vi "FGV_OBJ_error_buffer.vi"(4 "main_tab":refnum<vi>, 6 "thread":T1, 7 "option":T2=enum."display", 8 "error_in":errorcluster, 9 "error_indicator_global":refnum<vi>, 10 "error_indicator_tab":refnum<vi>, 11 "error_display_ref":refnum<vi>) -> (0 "error_out":errorcluster, 3 "error?":bool)   [LabVIEW 2020]
doc: "This VI check if error on error_in input is already in the buffer, and if not adds it to buffer and sends error event to event structure. VI also clears errors."
uses:
  FGV_OBJ_error_buffer.ctl
  MAIN/OBJ_thread.ctl
  <vilib>/Utility/miscctls.llb/LVRowAndColumnTypeDef.ctl
  <vilib>/Utility/miscctls.llb/LVRowAndColumnUnsignedTypeDef.ctl
  tristate_indicator_OBJ_test/FGV_tristate_indicator_OBJ_test.ctl
  _misc/AULocalize/SubVIs/Get Localized Phrase Compact Interface 1D.vi
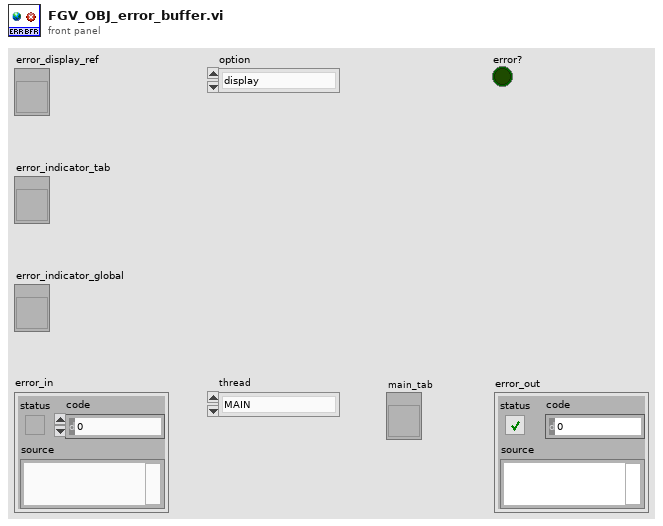
[diagram p1: front panel]
types:
  T1 = typedef "OBJ_thread.ctl" = enum16{"MAIN", "SCANNER", "MD - LEFT", "MD - RIGHT", "GUI TIMER"}
  T2 = typedef "FGV_OBJ_error_buffer.ctl" = enum16{"initialize", "clear", "display", "get_status"}
  T3 = typedef "LVRowAndColumnUnsignedTypeDef.ctl" = cluster{"Row":u32, "Column":u32}
  T4 = typedef "LVRowAndColumnTypeDef.ctl" = cluster{"Row":i32, "Column":i32}
  T5 = typedef "FGV_tristate_indicator_OBJ_test.ctl" = enum16{"initialize", "tooling", "ready", "pending", "OK", "NOK", "part_NOK", "routing_NOK", "repeat_NOK", "timeout", "translate", "error"}
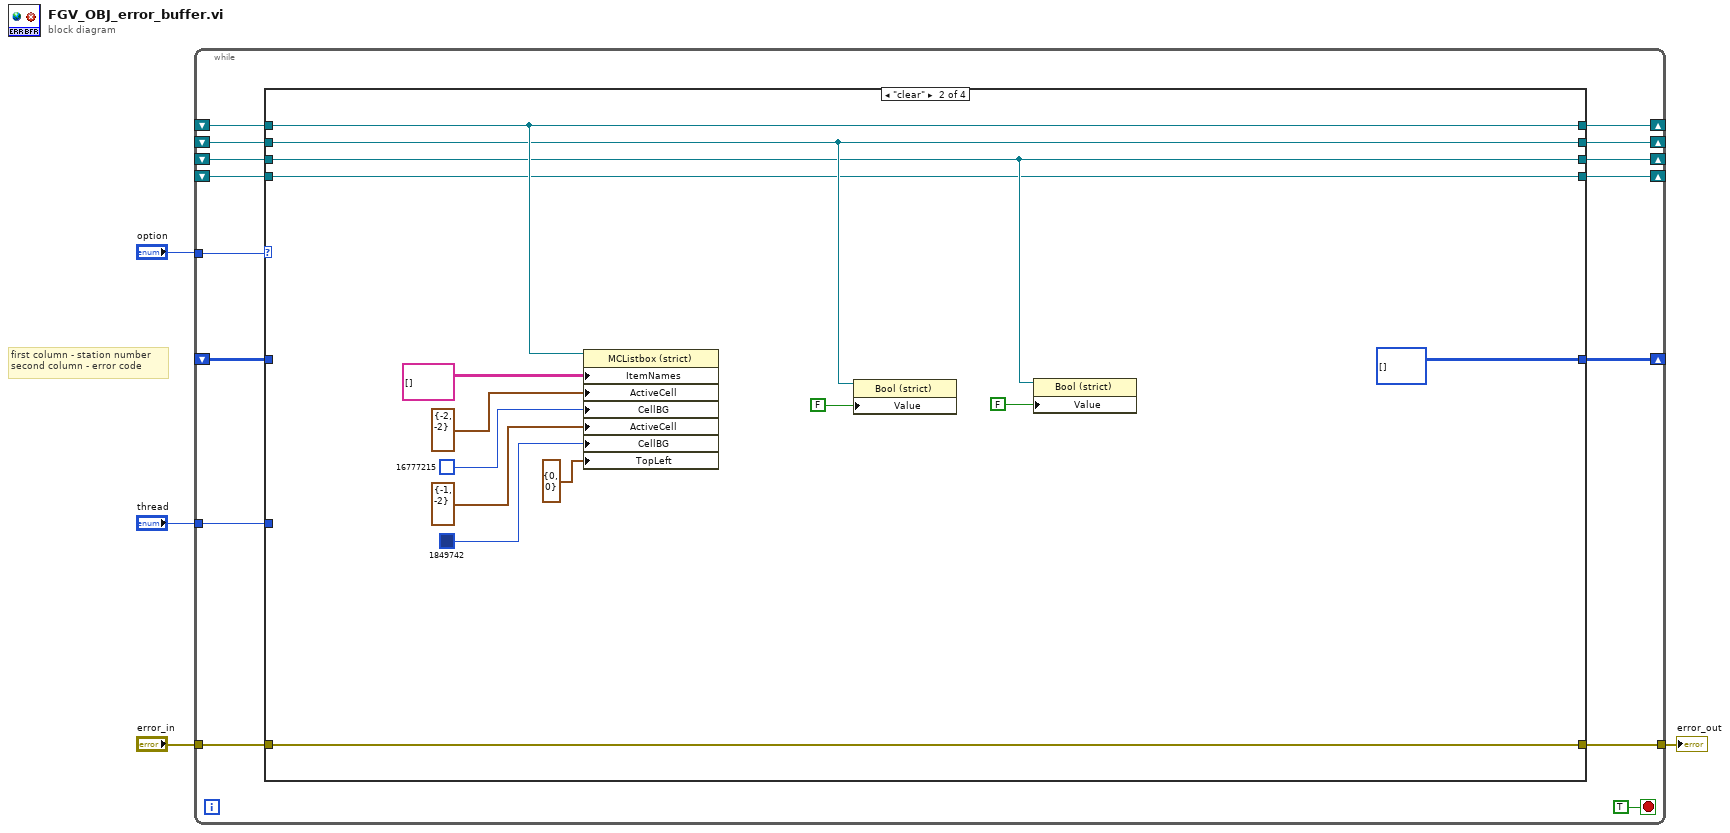
[diagram p0: block diagram]
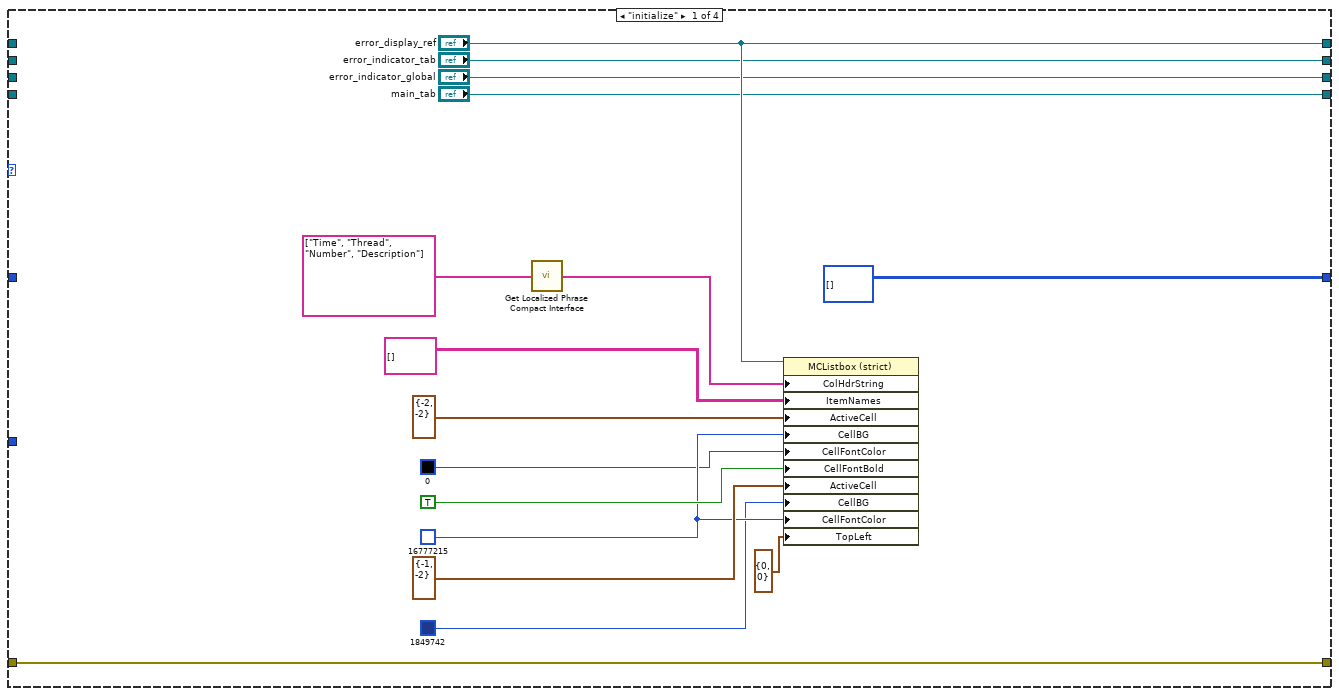
[diagram p2: hidden frame]
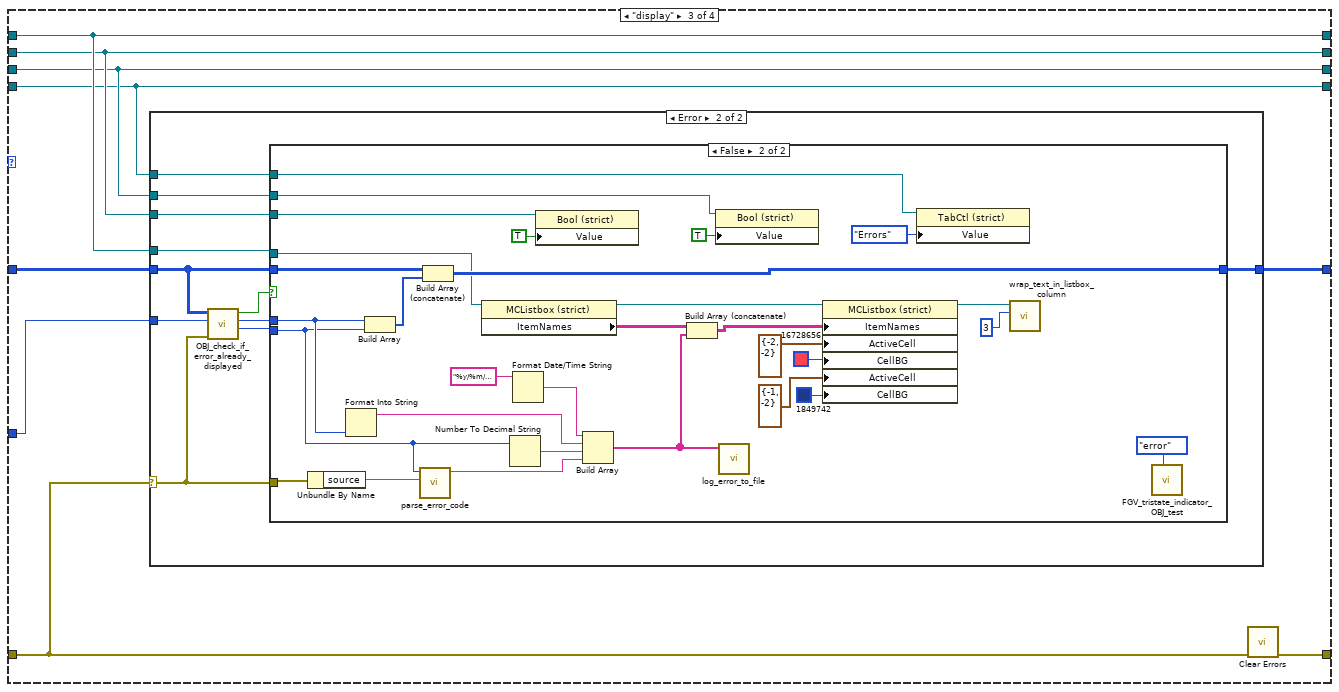
[diagram p3: hidden frame]
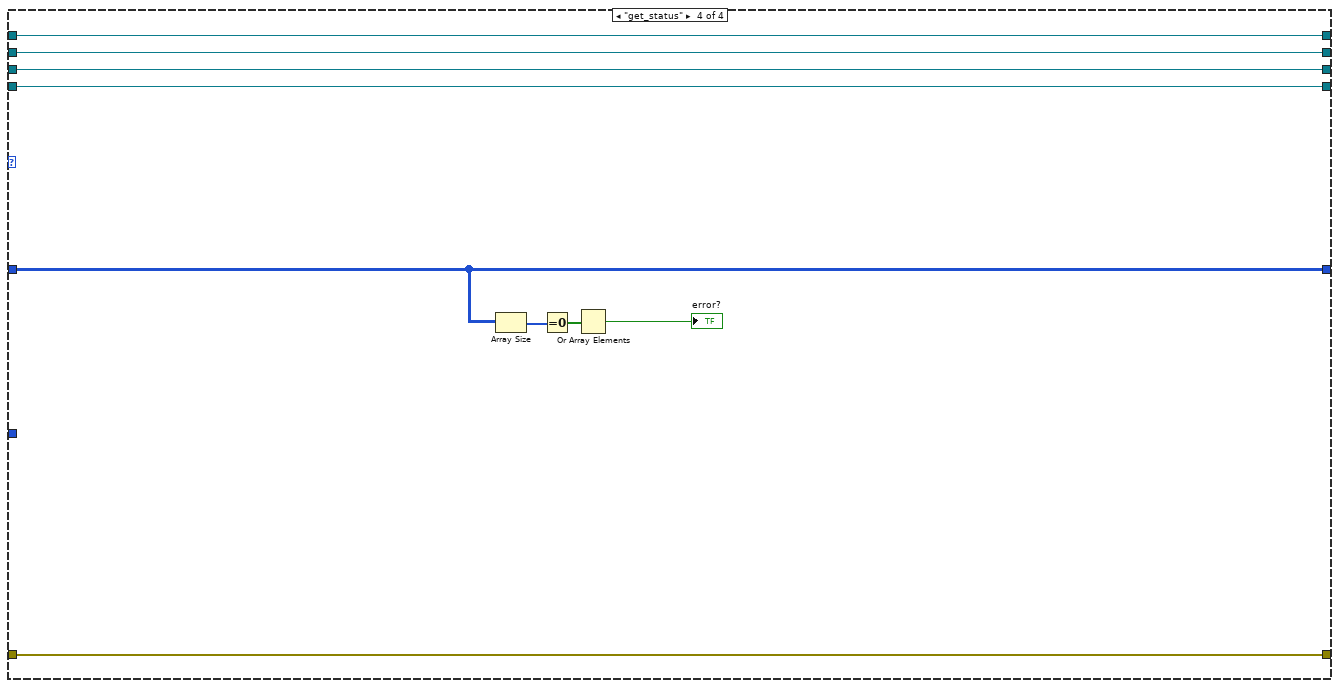
[diagram p6: hidden frame]
diagram:
  # "first column - station number\nsecond column - error code"
  n1 = while {
    tunnel: "option" -> [w18]
    tunnel: [w17] -> w4
    tunnel: "error_in" -> [w16]
    shift-right: [w15] -> _
    shift-left: _ -> [w14]
    shift-right: [w13] -> _
    shift-left: _ -> [w12]
    tunnel: "thread" -> [w11]
    shift-right: [w10] -> _
    shift-left: _ -> [w8]
    shift-right: [w9] -> _
    shift-left: _ -> [w7]
    shift-right: [w6] -> _
    shift-left: _ -> [w5]
    stop <- TRUE stop-if-true
    n2 = case shown="\"clear\"" w18 {
      tunnel: [w35 w49 w57 w109] -> w17
      tunnel: w16 -> [w35 w49 w56 w109]
      tunnel: [i32[][] [] i32[][] [] w55 w110] -> w15
      tunnel: w14 -> [_ _ w58 w110]
      tunnel: ["error_display_ref" w42 w53 w108] -> w13
      tunnel: w12 -> [_ w42 w53 w108]
      tunnel: w11 -> [_ _ w54 _]
      tunnel: ["error_indicator_tab" w41 w52 w104] -> w10
      tunnel: ["error_indicator_global" w40 w51 w103] -> w9
      tunnel: w8 -> [_ w41 w52 w104]
      tunnel: w7 -> [_ w40 w51 w103]
      tunnel: ["main_tab" w37 w50 w102] -> w6
      tunnel: w5 -> [_ w37 w50 w102]
      frame "initialize" {
        w31 = u32 16777215
        n3 = call-poly "Get Localized Phrase Compact Interface.vi"("Key"=string[] ["Time", "Thread", "Number", "Description"] ("Column Header Strings[]")) -> ("Translated Phrase"=w20:string[])
        n4 = property on="Property Node" class="MCListbox (strict)"(reference="error_display_ref", "ColHdrString"=w20, "ItemNames"=string[][] [] ("Item Names"), "ActiveCell"=T4 {"Row"=-2, "Column"=-2} ("Active Cell:Active Cell"), "CellBG"=w31, "CellFontColor"=u32 0, "CellFontBold"=TRUE ("Active Cell:Cell Font:Bold"), "ActiveCell"=T4 {"Row"=-1, "Column"=-2} ("Active Cell:Active Cell"), "CellBG"=u32 1849742, "CellFontColor"=w31, "TopLeft"=T3 {"Row"=0, "Column"=0} ("Top Left Visible Cell")) -> ()  [unwired: 1 in, 2 out]
      }
      frame "clear" {
        n5 = property on="Property Node" class="MCListbox (strict)"(reference=w42, "ItemNames"=string[][] [] ("Item Names"), "ActiveCell"=T4 {"Row"=-2, "Column"=-2} ("Active Cell:Active Cell"), "CellBG"=u32 16777215, "ActiveCell"=T4 {"Row"=-1, "Column"=-2} ("Active Cell:Active Cell"), "CellBG"=u32 1849742, "TopLeft"=T3 {"Row"=0, "Column"=0} ("Top Left Visible Cell")) -> ()  [unwired: 1 in, 2 out]
        n6 = property on="Property Node" class="Bool (strict)"(reference=w41, "Value"=FALSE) -> ()  [unwired: 1 in, 2 out]
        n7 = property on="Property Node" class="Bool (strict)"(reference=w40, "Value"=FALSE) -> ()  [unwired: 1 in, 2 out]
      }
      frame "display" {
        n8 = case shown="Error" w56 {
          selector: w56 -> [_ w64]
          tunnel: w58 -> [w59 w67]
          tunnel: [w59 w69] -> w55
          tunnel: w54 -> [_ w60]
          tunnel: w53 -> [_ w65]
          tunnel: w52 -> [_ w63]
          tunnel: w51 -> [_ w62]
          tunnel: w50 -> [_ w61]
          frame No Error {
          }
          frame Error {
            n9 = call "OBJ_check_if_error_already_displayed.vi"("error_in"=w64, "thread_in"=w60, "displayed_errors"=w67) -> ("error_code"=w66:i32, "thread_out"=w68:T1, "already_displayed?"=w70:bool)  [unwired: 6 in]
            n10 = case shown="False" w70 {
              tunnel: w67 -> [w71 w100]
              tunnel: [w71 w101] -> w69
              tunnel: w68 -> [_ w94]
              tunnel: w66 -> [_ w83]
              tunnel: w65 -> [_ w98]
              tunnel: w64 -> [_ w92]
              tunnel: w63 -> [_ w78]
              tunnel: w62 -> [_ w77]
              tunnel: w61 -> [_ w74]
              frame True {
              }
              frame False {
                n11 = Unbundle By Name(w92) -> ("source"=w84:string)
                n12 = Format Into String(w94) -> (resulting string=w93:string)  [unwired: 3 in, 1 out]
                n13 = Build Array(w94, w83) -> (w99:i32[])
                n14 = call "parse_error_code.vi"("source"=w84, "code"=w83) -> ("parsed_error_string"=w82:string)  [unwired: 9 in]
                n15 = Build Array (concatenate)(w100, w99) -> (w101:i32[][])
                n16 = property class="MCListbox (strict)"(reference=w98) -> (reference out=w86:refnum<vi>, "ItemNames"=w91:string[][])  [unwired: 1 in, 1 out]
                n17 = Number To Decimal String(number=w83) -> (decimal integer string=w95:string)  [unwired: 1 in]
                n18 = Format Date/Time String(time format string (%c)="%y/%m/%d %H:%M:%S") -> (date/time string=w97:string)  [unwired: 2 in]
                n19 = property on="Property Node" class="Bool (strict)"(reference=w78, "Value"=TRUE) -> ()  [unwired: 1 in, 2 out]
                n20 = Build Array(w97, w93, w95, w82) -> (w81:string[])
                n21 = Build Array (concatenate)(w91, w81) -> (w85:string[][])
                n22 = property on="Property Node" class="Bool (strict)"(reference=w77, "Value"=TRUE) -> ()  [unwired: 1 in, 2 out]
                n23 = call "log_error_to_file.vi"("error_info"=w81) -> ()  [unwired: 11 in]
                n24 = property on="Property Node" class="MCListbox (strict)"(reference=w86, "ItemNames"=w85, "ActiveCell"=T4 {"Row"=-2, "Column"=-2} ("Active Cell:Active Cell"), "CellBG"=u32 16728656 ("Color Box"), "ActiveCell"=T4 {"Row"=-1, "Column"=-2} ("Active Cell:Active Cell"), "CellBG"=u32 1849742) -> (reference out=w76:refnum<vi>)  [unwired: 1 in, 1 out]
                n25 = property on="Property Node" class="TabCtl (strict)"(reference=w74, "Value"=enum32{"OBJ Test", "Errors"}."Errors") -> ()  [unwired: 1 in, 2 out]
                n26 = call "wrap_text_in_listbox_column.vi"("colum_to_wrap"=3, "multicolumn_listbox_reference"=w76) -> ()  [unwired: 8 in, 2 out]
                n27 = call "FGV_tristate_indicator_OBJ_test.vi"("options"=FGV_tristate_indicator_OBJ_test."error") -> ()  [unwired: 10 in, 1 out]
              }
            }
          }
        }
        n28 = call <vilib>:"Clear Errors.vi"("error in (no error)"=w56) -> ("error out"=w57:errorcluster)  [unwired: 5 in, 1 out]
      }
      frame "get_status" {
        n29 = Array Size(array=w110) -> (size(s)=w107:i32[])
        n30 = Equal To 0?(x=w107) -> (x = 0?=w106:bool[])
        n31 = Or Array Elements(Boolean array=w106) -> (logical OR=→"error?":bool)
      }
    }
  }
  "error_out" <- w4
